vi "Read Frame (using FPGA) (SubVI).vi"(10 "Data In":T1={"Image Height"=3072, "Image Width"=3072, "Frame Rate"=3072, "Movie File REF"=refnum, "Image REF"=refnum, "FPGA REF"=refnum}) -> (0 "EOF":bool, 1 "Image Data":u64[](array[numeric]), 3 "Frame Number":u64)   [LabVIEW 2015]
uses:
  Controls (HOST)/Replay Data Bundle.ctl
  <vilib>/vision/Image Controls.llb/IMAQ Image.ctl
  <vilib>/Utility/error.llb/Error Cluster From Error Code.vi
  <vilib>/rvi/errors/niLvFpgaAdjustHostInterfaceError.vi
  <vilib>/rvi/interface/nirviMethod/nirviMethod.xnode
  <vilib>/FPGAPlugInAG/Dynamic/niLvFpga_WriteFifo_Dynamic.vi
  <vilib>/rvi/errors/niLvFpgaMergeErrorWithErrorCode.vi
  <vilib>/FPGAPlugInAG/Dynamic/niLvFpga_ReadFifo_Dynamic.vi
panel:
  out "File REF Out":refnum<file>
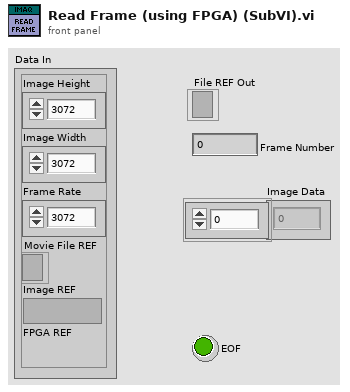
[diagram p1: front panel]
types:
  T1 = typedef "Replay Data Bundle.ctl" = cluster{"Image Height":i32, "Image Width":i32, "Frame Rate":i32, "Movie File REF":refnum<file>, "Image REF":T2, "FPGA REF":refnum<k20>}
  T2 = typedef "IMAQ Image.ctl" = refnum<image>
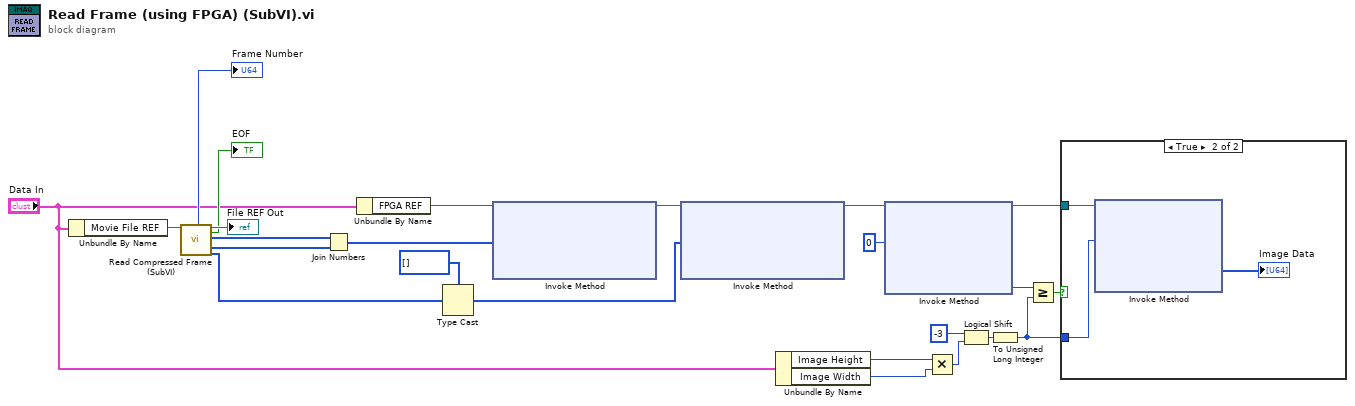
[diagram p0: block diagram]
diagram:
  n1 = Unbundle By Name("Data In") -> ("Movie File REF"=w7:refnum<file>)
  n2 = call "Read Compressed Frame (SubVI).vi"("File REF In"=w7) -> ("Frame Number"=→"Frame Number":u64, "File REF Out"=→"File REF Out":refnum<file>, "EOF"=→"EOF":bool, "Bit Depth"=w10:u8[], "Minimum"=w9:u8[], "Data"=w8:u8[])  [unwired: 12 in, 1 out]
  n3 = Join Numbers(hi=w10, lo=w9) -> ((hi.lo)=w11:u16[])
  n4 = Unbundle By Name("Data In") -> ("FPGA REF"=w24:refnum<k20>)
  n5 = Type Cast(type=u64[] [] ("output array"), x=w8) -> (*(type *) &x=w1:u64[])
  n6 = xnode "Invoke Method"("FPGA VI Reference In"=w24, "Data"=w11) -> ("FPGA VI Reference Out"=w3:refnum<k20>)  [unwired: 2 in, 2 out]
  n7 = xnode "Invoke Method"("FPGA VI Reference In"=w3, "Data"=w1) -> ("FPGA VI Reference Out"=w17:refnum<k20>)  [unwired: 2 in, 2 out]
  n8 = Unbundle By Name("Data In") -> ("Image Height"=w4:i32, "Image Width"=w5:i32)
  n9 = xnode "Invoke Method"("FPGA VI Reference In"=w17, "Number of Elements"=u32 0) -> ("FPGA VI Reference Out"=w15:refnum<k20>, "Elements Remaining"=w19:u32)  [unwired: 2 in, 2 out]
  n10 = Multiply(x=w4, y=w5) -> (x*y=w23:i32)
  n11 = Logical Shift(y=i16 -3, x=w23) -> (x << y=w21:i32)
  n12 = To Unsigned Long Integer(number=w21) -> (unsigned 32bit integer=w18:u32)
  n13 = Greater Or Equal?(x=w19, y=w18) -> (x >= y?=w16:bool)
  n14 = case shown="True" w16 {
    tunnel: w18 -> [_ w27]
    tunnel: w15 -> [_ w26]
    frame False {
    }
    frame True {
      n15 = xnode "Invoke Method"("FPGA VI Reference In"=w26, "Number of Elements"=w27) -> ("Data"=→"Image Data":u64[])  [unwired: 2 in, 3 out]
    }
  }
